vi "getCamera2.vi"(8 "error in (no error)":errorcluster, 11 "HWConfiguration.lvclass in":refnum<class "HWConfiguration.lvclass">) -> (0 "error out":errorcluster, 2 "camera2":string, 3 "HWConfiguration.lvclass out":refnum<class "HWConfiguration.lvclass">)   [LabVIEW 2011, in "Hardware.lvlib" / "HWControllers.lvlib" / "HWConfiguration.lvclass"]
doc: "Which Camera is in use?"
uses:
  HWConfiguration.lvclass
  HWConfiguration.lvclass/HWConfiguration.ctl
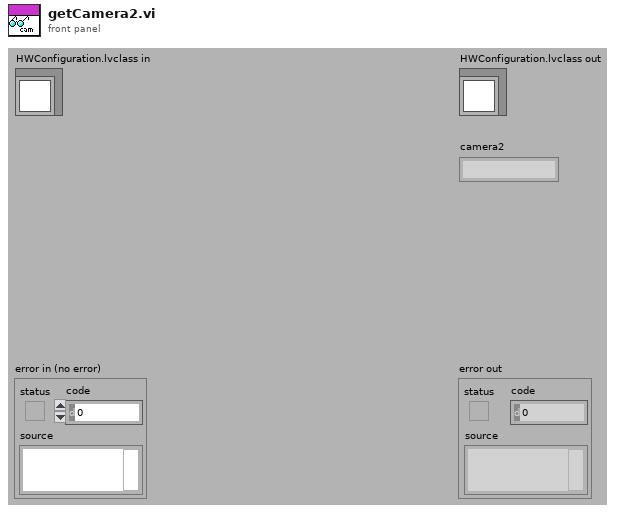
[diagram p1: front panel]
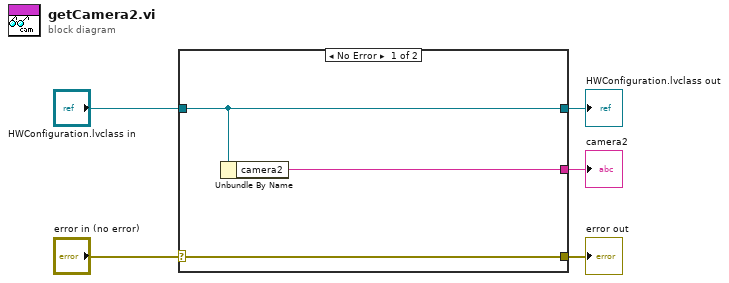
[diagram p0: block diagram]
diagram:
  n1 = case shown="No Error" "error in (no error)" {
    selector: "error in (no error)" -> [w8 w9]
    tunnel: [w8 w9] -> w4
    tunnel: [w7 w10] -> w2
    tunnel: "HWConfiguration.lvclass in" -> [w7 w10]
    tunnel: [w6 _] -> w1
    frame No Error {
      n2 = Unbundle By Name(w7) -> ("camera2"=w6:string)
    }
    frame Error {
    }
  }
  "error out" <- w4
  "HWConfiguration.lvclass out" <- w2
  "camera2" <- w1
